vi "Color-Senser-Read_Test.vi"() -> ()   [LabVIEW 2019]
panel:
  in  "觸發數值":dbl=90.0 format="%#_13g"
  out "當前數值":dbl
  out "觸發?":bool
  out "Error Out":errorcluster
  in  "Error In":errorcluster
  in  "Stop":bool
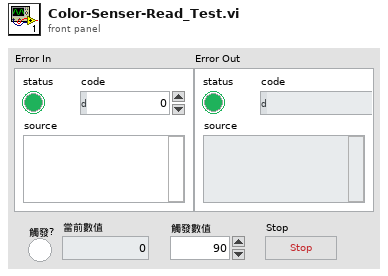
[diagram p1: front panel]
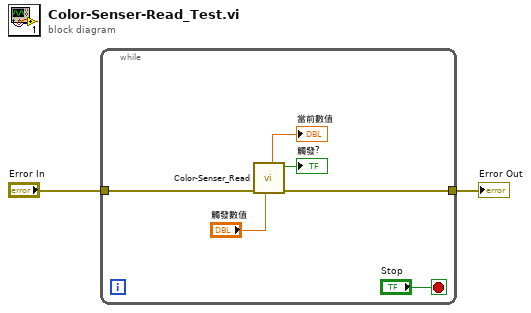
[diagram p0: block diagram]
diagram:
  n1 = while {
    tunnel: "Error In" -> [w7]
    tunnel: [w6] -> w1
    stop <- "Stop" stop-if-true
    n2 = call "Color-Senser_Read.vi"("觸發數值"="觸發數值", "Error In"=w7) -> ("Error Out"=w6:errorcluster, "觸發?"=→"觸發?":bool, "當前數值"=→"當前數值":dbl)  [unwired: 7 in]
  }
  "Error Out" <- w1
